vi "图片切换.vi"() -> ()   [LabVIEW 2018]
panel:
  out "下拉列表":u16(ring)
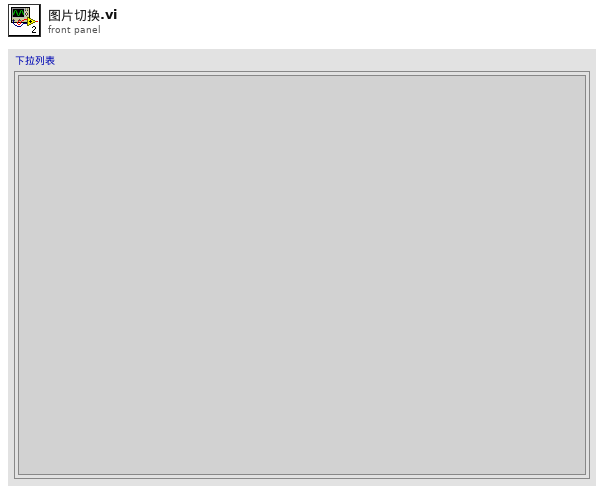
[diagram p1: front panel]
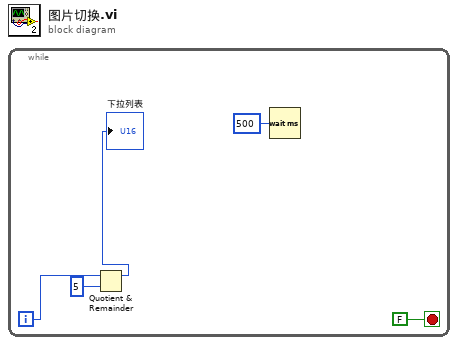
[diagram p0: block diagram]
diagram:
  n1 = while {
    i -> [w3]
    stop <- FALSE stop-if-true
    n2 = Quotient & Remainder(x=w3, y=5) -> (x-y*floor(x/y)=→"下拉列表":i32)  [unwired: 1 out]
    n3 = Wait (ms)(milliseconds to wait=u32 500 ("等待时间（毫秒）")) -> ()  [unwired: 1 out]
  }
